vi "MGCC_MdlMgmt_Topology.vi"() -> ()   [LabVIEW 2016]
doc: "This VI is designed to initize the SHE215 model with topology (2D double array)."
uses:
  <vilib>/imath/engines/lvmath2/RunTimeEngine/NodeEndStatement/NIMS_NodeEndStatement_Output.vi
  <instcachedir>/0/NIMS_NodeEndStatement_Output_53EC0D466D134D7ABD903AC30B43404B.lvgen/NIMS_NodeEndStatement_Output_53EC0D466D134D7ABD903AC30B43404B_002.vi
  <vilib>/imath/engines/lvmath2/RunTimeEngine/ErrorHandling/NIMS_Finalize Error.vi
panel:
  out "array":dbl[][](array[numeric])
  out "text":string
  out "Topology":dbl[][](array[numeric])
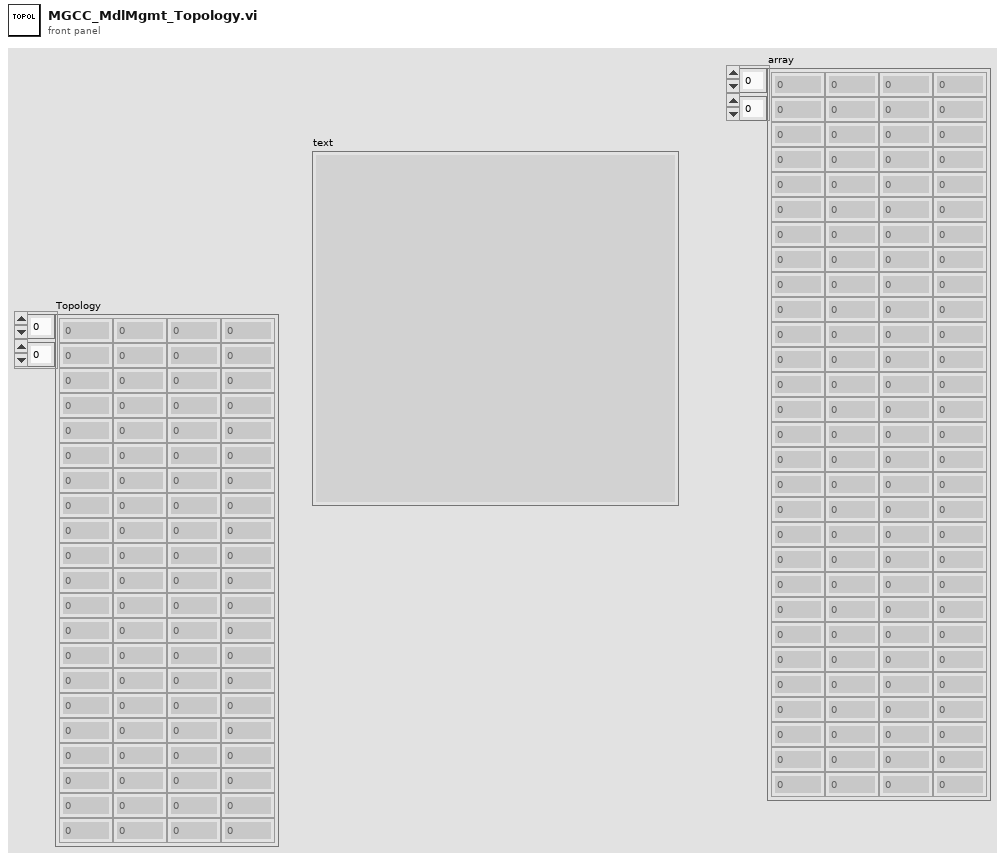
[diagram p1: front panel]
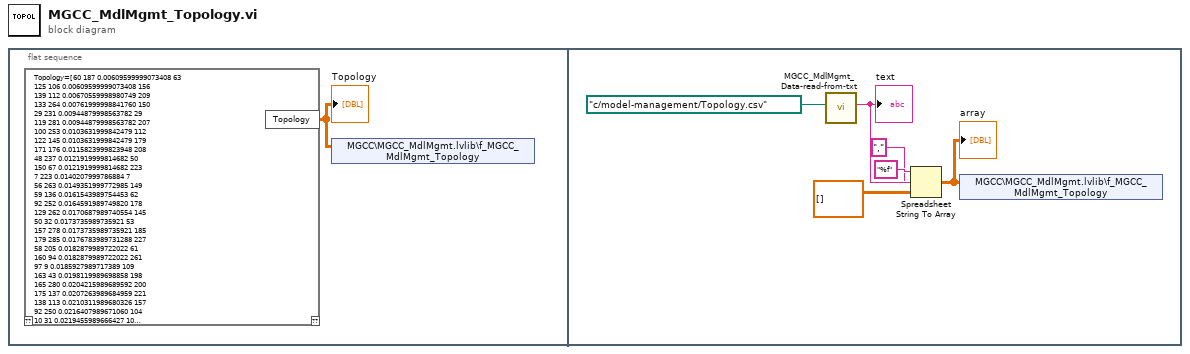
[diagram p0: block diagram]
diagram:
  n1 = flat-sequence {
    frame #0 {
      n2 = mathscript code="Topology=[60\t187\t0.00609599999073408\t63\n125\t106\t0.00609599999073408\t156\n139\t112\t0.00670559998980749\t209\n133\t264\t0.00761999998841760\t150\n29\t231\t0.00944879998563782\t29\n119\t281\t0.00944879998563782\t207\n100\t253\t0.0103631999842479\t112\n122\t145\t0.0103631999842479\t179\n171\t176\t0.0115823999823948\t208\n48\t237\t0.0121919999814682\t50\n150\t67\t0.0121919999814682\t223\n7\t223\t0.0140207999786884\t7\n56\t263\t0.0149351999772985\t149\n59\t136\t0.0161543989754453\t62\n92\t252\t0.0164591989749820\t178\n129\t262\t0.0170687989740554\t145\n50\t32\t0.0173735989735921\t53\n157\t278\t0.0173735989735921\t185\n179\t285\t0.0176783989731288\t227\n58\t205\t0.0182879989722022\t61\n160\t94\t0.0182879989722022\t261\n97\t9\t0.0185927989717389\t109\n163\t43\t0.0198119989698858\t198\n165\t280\t0.0204215989689592\t200\n175\t137\t0.0207263989684959\t221\n138\t113\t0.0210311989680326\t157\n92\t250\t0.0216407989671060\t104\n10\t31\t0.0219455989666427\t10\n96\t149\t0.0219455989666427\t151\n25\t228\t0.0222503989661794\t25\n202\t96\t0.0225551989657161\t266\n199\t239\t0.0231647989647895\t255\n49\t76\t0.0234695989643262\t52\n4\t44\t0.0234695989643262\t100\n16\t23\t0.0237743989638629\t42\n52\t239\t0.0237743989638629\t55\n61\t179\t0.0237743989638629\t212\n114\t68\t0.0243839989629363\t128\n154\t86\t0.0243839989629363\t192\n125\t178\t0.0246887989624730\t141\n167\t157\t0.0246887989624730\t202\n80\t287\t0.0246887989624730\t231\n146\t191\t0.0252983989615464\t170\n37\t193\t0.0252983989615464\t191\n43\t235\t0.0256031989610831\t44\n184\t190\t0.0256031989610831\t238\n214\t57\t0.0256031989610831\t287\n15\t144\t0.0259079989606198\t260\n205\t294\t0.0262127989601565\t269\n65\t93\t0.0265175989596933\t70\n151\t276\t0.0271271989587667\t176\n198\t88\t0.0271271989587667\t254\n83\t152\t0.0274319989583034\t93\n107\t142\t0.0274319989583034\t120\n190\t268\t0.0277367989578401\t245\n194\t90\t0.0280415989573768\t250\n124\t74\t0.0283463989569135\t140\n43\t283\t0.0283463989569135\t219\n75\t71\t0.0289559989559869\t83\n136\t265\t0.0289559989559869\t154\n61\t148\t0.0292607989555236\t278\n80\t246\t0.0298703989545970\t88\n91\t249\t0.0298703989545970\t103\n108\t175\t0.0298703989545970\t121\n19\t69\t0.0301751989541337\t19\n121\t46\t0.0301751989541337\t135\n111\t82\t0.0304799989536704\t138\n173\t282\t0.0304799989536704\t217\n111\t257\t0.0307847989532071\t124\n113\t143\t0.0307847989532071\t127\n104\t36\t0.0310895989527438\t117\n117\t183\t0.0313943989522805\t131\n122\t261\t0.0313943989522805\t137\n112\t258\t0.0316991989518172\t126\n150\t275\t0.0326135989504273\t175\n154\t272\t0.0329183989499640\t182\n54\t102\t0.0335279989490374\t57\n183\t158\t0.0335279989490374\t237\n53\t97\t0.0338327989485742\t56\n23\t170\t0.0338327989485742\t75\n81\t199\t0.0338327989485742\t89\n13\t101\t0.0341375989481109\t92\n218\t129\t0.0341375989481109\t292\n149\t7\t0.0344423989476476\t173\n208\t65\t0.0344423989476476\t279\n20\t128\t0.0347471989471843\t20\n73\t32\t0.0347471989471843\t81\n90\t160\t0.0347471989471843\t216\n163\t130\t0.0347471989471843\t235\n215\t166\t0.0347471989471843\t288\n23\t227\t0.0350519989467210\t23\n28\t29\t0.0350519989467210\t28\n144\t196\t0.0350519989467210\t271\n96\t139\t0.0353567989462577\t108\n54\t117\t0.0359663989453311\t90\n87\t208\t0.0362711989448678\t98\n36\t206\t0.0365759989444045\t36\n20\t236\t0.0365759989444045\t47\n189\t290\t0.0365759989444045\t244\n74\t148\t0.0368807989439412\t82\n181\t72\t0.0368807989439412\t264\n108\t12\t0.0374903989430146\t229\n128\t87\t0.0377951989425513\t144\n144\t271\t0.0377951989425513\t168\n196\t292\t0.0377951989425513\t252\n102\t107\t0.0380999989420880\t115\n170\t47\t0.0380999989420880\t205\n2\t21\t0.0384047989416247\t2\n39\t132\t0.0384047989416247\t222\n7\t28\t0.0390143989406981\t51\n134\t53\t0.0393191989402348\t152\n220\t240\t0.0393191989402348\t296\n35\t100\t0.0396239989397715\t35\n156\t116\t0.0396239989397715\t184\n204\t120\t0.0396239989397715\t268\n206\t35\t0.0396239989397715\t273\n123\t171\t0.0399287989393082\t139\n193\t291\t0.0402335989388449\t249\n26\t260\t0.0405383989383816\t242\n192\t159\t0.0405383989383816\t248\n94\t201\t0.0408431989379183\t106\n114\t257\t0.0411479989374550\t159\n176\t134\t0.0411479989374550\t224\n135\t181\t0.0414527989369917\t153\n148\t273\t0.0414527989369917\t172\n45\t270\t0.0414527989369917\t293\n16\t138\t0.0417575989365284\t16\n159\t51\t0.0417575989365284\t188\n46\t126\t0.0420623989360652\t48\n162\t99\t0.0420623989360652\t196\n210\t135\t0.0420623989360652\t282\n22\t60\t0.0423671989356019\t22\n93\t295\t0.0423671989356019\t274\n78\t100\t0.0429767989346753\t86\n41\t104\t0.0432815989342120\t41\n221\t232\t0.0432815989342120\t298\n51\t238\t0.0435863989337487\t54\n6\t95\t0.0441959989328221\t6\n79\t156\t0.0441959989328221\t87\n145\t272\t0.0445007989323588\t169\n166\t140\t0.0448055989318955\t201\n204\t89\t0.0448055989318955\t270\n27\t230\t0.0451103989314322\t27\n32\t18\t0.0457199989305056\t32\n139\t269\t0.0457199989305056\t162\n8\t224\t0.0466343989291157\t8\n22\t127\t0.0472439979281891\t297\n140\t192\t0.0475487979277258\t164\n155\t213\t0.0478535979272625\t257\n56\t34\t0.0481583979267992\t59\n137\t266\t0.0481583979267992\t155\n94\t2\t0.0484631979263359\t190\n181\t286\t0.0484631979263359\t230\n151\t279\t0.0484631979263359\t232\n124\t49\t0.0484631979263359\t263\n150\t85\t0.0484631979263359\t272\n76\t245\t0.0490727979254093\t84\n142\t25\t0.0490727979254093\t166\n182\t288\t0.0490727979254093\t233\n11\t240\t0.0496823979244828\t64\n132\t161\t0.0496823979244828\t148\n213\t210\t0.0502919979235562\t286\n33\t203\t0.0505967979230929\t33\n164\t279\t0.0505967979230929\t199\n203\t59\t0.0505967979230929\t267\n82\t8\t0.0509015979226296\t91\n188\t155\t0.0512063979221663\t243\n118\t191\t0.0515111979217030\t132\n119\t260\t0.0518159979212397\t133\n160\t12\t0.0521207979207764\t193\n67\t189\t0.0524255979203131\t72\n126\t218\t0.0524255979203131\t142\n13\t219\t0.0527303979198498\t13\n143\t164\t0.0530351979193865\t167\n106\t79\t0.0536447979184599\t119\n115\t195\t0.0539495979179966\t129\n201\t58\t0.0539495979179966\t259\n127\t209\t0.0542543979175333\t143\n130\t1\t0.0545591979170700\t146\n158\t80\t0.0545591979170700\t187\n120\t254\t0.0548639979166067\t215\n169\t133\t0.0551687979161434\t204\n174\t243\t0.0557783979152168\t218\n77\t198\t0.0560831979147535\t85\n49\t243\t0.0563879979142902\t79\n52\t202\t0.0563879979142902\t160\n52\t5\t0.0563879979142902\t197\n105\t89\t0.0566927979138270\t125\n147\t78\t0.0569975979133637\t171\n103\t27\t0.0569975979133637\t236\n61\t197\t0.0579119979119738\t65\n42\t194\t0.0579119979119738\t211\n15\t215\t0.0582167979115105\t246\n15\t115\t0.0591311979101206\t15\n5\t11\t0.0594359979096573\t5\n93\t251\t0.0594359979096573\t105\n11\t131\t0.0597407979091940\t11\n69\t17\t0.0597407979091940\t74\n59\t198\t0.0597407979091940\t206\n10\t84\t0.0597407979091940\t213\n94\t284\t0.0600455979087307\t220\n148\t56\t0.0600455979087307\t234\n14\t225\t0.0603503979082674\t14\n31\t102\t0.0603503979082674\t31\n85\t141\t0.0603503979082674\t96\n95\t214\t0.0603503979082674\t107\n4\t222\t0.0606551979078041\t4\n55\t14\t0.0609599979073408\t58\n4\t174\t0.0609599979073408\t163\n5\t268\t0.0612647979068775\t161\n141\t270\t0.0612647979068775\t165\n161\t75\t0.0612647979068775\t195\n17\t121\t0.0615695979064142\t17\n34\t19\t0.0618743979059509\t34\n45\t55\t0.0618743979059509\t46\n195\t4\t0.0618743979059509\t251\n109\t221\t0.0624839979050243\t122\n209\t169\t0.0627887979045610\t281\n219\t299\t0.0640079979027078\t295\n9\t23\t0.0646175979017813\t9\n71\t15\t0.0646175979017813\t78\n89\t247\t0.0646175979017813\t101\n131\t245\t0.0646175979017813\t147\n180\t163\t0.0649223979013179\t262\n169\t290\t0.0649223979013179\t277\n39\t233\t0.0658367978999281\t39\n90\t248\t0.0667511978985382\t102\n84\t20\t0.0670559978980749\t95\n86\t110\t0.0670559978980749\t97\n47\t204\t0.0673607978976116\t49\n50\t126\t0.0673607978976116\t214\n116\t259\t0.0685799978957584\t130\n1\t119\t0.0691895978948318\t1\n137\t267\t0.0694943978943685\t158\n73\t114\t0.0704087978929786\t94\n57\t182\t0.0707135978925153\t60\n202\t296\t0.0707135978925153\t283\n27\t3\t0.0719327978906622\t181\n185\t214\t0.0719327978906622\t239\n103\t207\t0.0728471978892723\t136\n72\t244\t0.0731519978888090\t80\n187\t186\t0.0731519978888090\t241\n186\t289\t0.0737615978878824\t240\n197\t109\t0.0740663978874191\t253\n44\t188\t0.0743711978869558\t45\n103\t30\t0.0746759978864925\t116\n37\t232\t0.0755903978851026\t37\n62\t9\t0.0755903978851026\t66\n168\t6\t0.0755903978851026\t203\n18\t98\t0.0777239978818595\t18\n98\t38\t0.0777239978818595\t110\n26\t229\t0.0780287978813962\t26\n42\t234\t0.0783335968809329\t43\n116\t91\t0.0783335968809329\t280\n70\t167\t0.0786383968804696\t76\n40\t36\t0.0789431968800063\t40\n88\t151\t0.0810767968767633\t99\n21\t226\t0.0813815968763000\t21\n120\t64\t0.0819911968753734\t134\n45\t185\t0.0822959968749101\t189\n22\t48\t0.0826007968744468\t77\n167\t26\t0.0826007968744468\t275\n211\t37\t0.0832103968735202\t284\n175\t211\t0.0841247968721303\t294\n64\t91\t0.0883919968656442\t68\n177\t162\t0.0908303968619378\t225\n12\t41\t0.0914399968610112\t12\n101\t255\t0.0914399968610112\t114\n61\t10\t0.0917447968605479\t69\n20\t70\t0.0917447968605479\t258\n27\t153\t0.0926591968591580\t186\n191\t62\t0.0926591968591580\t247\n99\t252\t0.0929639968586947\t111\n42\t254\t0.0935735968577681\t113\n38\t216\t0.0950975968554517\t38\n216\t297\t0.0957071968545251\t289\n105\t256\t0.0960119968540618\t118\n180\t101\t0.0966215968531352\t228\n118\t274\t0.0978407968512820\t174\n66\t173\t0.0984503968503554\t71\n99\t229\t0.0987551968498921\t194\n155\t277\t0.103936796842016\t183\n63\t241\t0.106679996837846\t67\n207\t177\t0.108813596834603\t276\n68\t242\t0.109118396834140\t73\n3\t217\t0.110642395831824\t3\n173\t212\t0.111556795830434\t291\n212\t8\t0.112166395829507\t285\n153\t186\t0.118871995819315\t180\n30\t165\t0.119481595818388\t30\n200\t172\t0.124358395810975\t256\n146\t293\t0.127406395806342\t265\n110\t200\t0.130759195801246\t123\n217\t298\t0.130759195801246\t290\n172\t24\t0.147523194775765\t210\n152\t63\t0.181660793723876\t177\n24\t83\t0.197205593700247\t24\n178\t261\t0.340766388482035\t226];"() -> ("Topology"=w1:dbl[][])  [unwired: 1 in, 1 out]
      "Topology" <- w1
      n3 = shared-variable "MGCC\\MGCC_MdlMgmt.lvlib\\f_MGCC_MdlMgmt_Topology"(w1) -> ()  [unwired: 1 in, 1 out]
    }
    frame #1 {
      n4 = call "MGCC_MdlMgmt_Data-read-from-txt.vi"("file path (use dialog)"=path "c:/model-management/Topology.csv") -> ("text"=w19:string)  [unwired: 10 in]
      "text" <- w19
      n5 = Spreadsheet String To Array(delimiter (Tab)=",", format string="%f", spreadsheet string=w19, array type (2D Dbl)=dbl[][] []) -> (array=w15:dbl[][])
      "array" <- w15
      n6 = shared-variable "MGCC\\MGCC_MdlMgmt.lvlib\\f_MGCC_MdlMgmt_Topology"(w15) -> ()  [unwired: 1 in, 1 out]
    }
  }
